vi "Validate Against JSON Schema.vi"(7 "JSON Schema":string="{\"type\": \"object\",\n\"required\":[\"Str\"],\n  \"properties\": {\n    \"Str\": { \"type\": \"string\"},\n    \"Num\": { \"type\": \"number\"}\n    }\n}", 8 "error in (no error)":errorcluster, 10 "Offset (JSON)":i32, 11 "JSON":string="{\"Str\":\"abc\",\n\"Numb\":123.456,\n\"Int\":123\n}") -> (0 "error out":errorcluster, 1 "<JSON>Failed Test":string, 2 "Path to Failed Test":string, 3 "Invalid":bool, 4 "<JSON>Failed SubJSON":string)   [LabVIEW 2021, in "json.facade.lvlib"]
doc: "Validate JSON versus a JSON Schema: https://json-schema.org/understanding-json-schema\n\nImpliments the following key words of JSON Schema:\n <b>\"type\", \"enum\", \"const\", \"allOf\", \"anyOf\", \"oneOf\", \"not\", \"if\", \"then\", \"else\"</b>\n Extra words for different JSON types:\n JSON Object: <b>\"properties\", \"required\", \"additionalProperties\",\"propertyNames\"</b>\n JSON Array: <b>\"prefixItems\", \"items\" (or \"additionalItems\"), \"minItems\", \"maxItems</b>\n String: <b>\"minLength\", \"maxLength\", \n <b>\"pattern\"</b> (uses LabVIEW inbuilt RegEx), \n <b>\"format\"</b> (only \"date-time\" implimented)\n Number: <b>minimum, maximum, exclusiveMinimum, exclusiveMaximum</b>\n\nIf the JSON Schema test fails, then \"Invalid\" will return True, \"Path to Failed Test\" will be a JSONpath pointer to the failed test, and \"Failed SubJSON\" will be a section of teh JSON that failed the test."
uses:
  json.facade.lvlib
  jsontext/JSONtext.lvlib
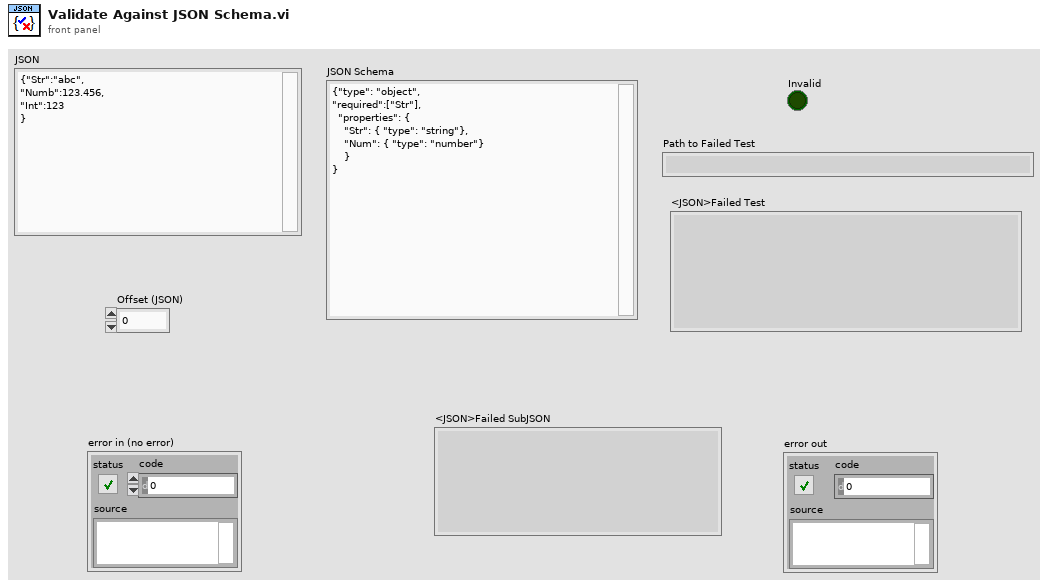
[diagram p1: front panel]
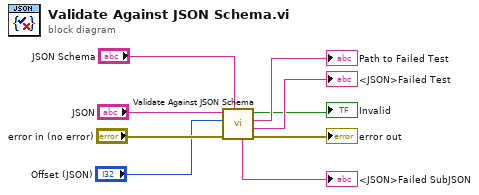
[diagram p0: block diagram]
diagram:
  n1 = call "Validate Against JSON Schema.vi"("JSON Schema"="JSON Schema", "error in (no error)"="error in (no error)", "Offset (JSON)"="Offset (JSON)", "JSON"="JSON") -> ("error out"=→"error out":errorcluster, "<JSON>Failed Test"=→"<JSON>Failed Test":string, "Path to Failed Test"=→"Path to Failed Test":string, "Invalid"=→"Invalid":bool, "<JSON>Failed SubJSON"=→"<JSON>Failed SubJSON":string)  [unwired: 3 in]
